vi "traffic control controller.vi"(0 "Is Logging":T3(array[cluster]), 1 "State":u16(ring) items=["Init", "Write"], 5 "Avalanch Packets":T2(array[cluster]) {"A1 std" format="%.1f"; "A2 std" format="%.1f"; "A3 std" format="%.1g"; "A4 std" format="%.1g"}, 13 "Trafikkontroll terskelverdier":T1(array[cluster])) -> (4 "Rød mast":bool[](array[boolean]), 10 "num pack rød lys i sekvens":u16[](array[numeric]), 14 "Is Logging":bool[](array[boolean]))   [LabVIEW 2017]
panel:
  out "num pack rød lys i totalt":u16[](array[numeric])
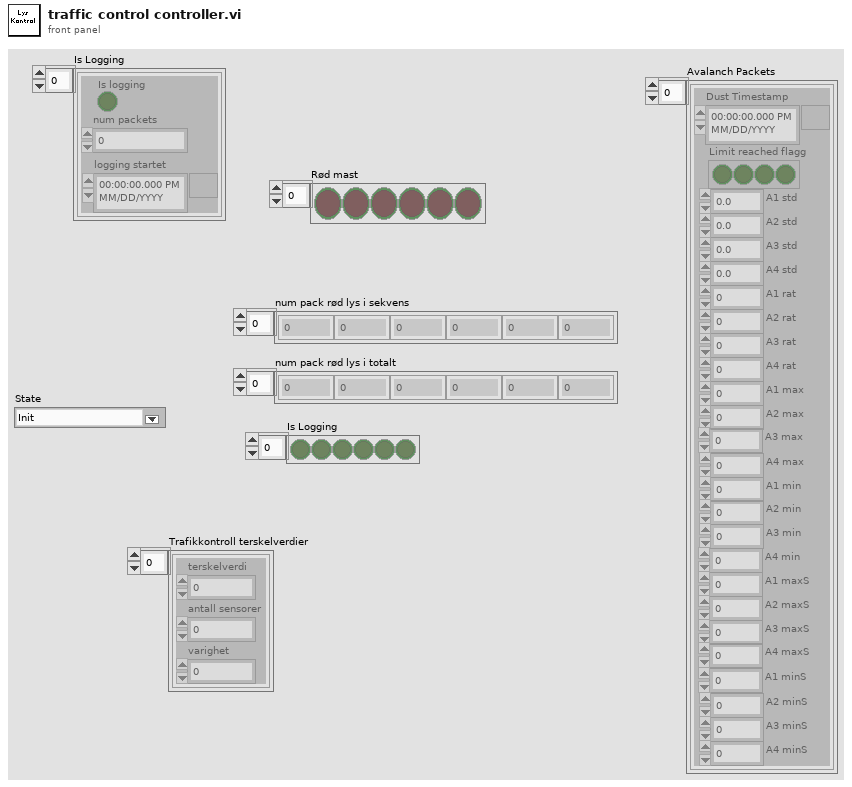
[diagram p1: front panel]
types:
  T1 = cluster{"terskelverdi":u32, "antall sensorer":u32, "varighet":u32}[]
  T2 = cluster{"Dust Timestamp":timestamp, "Limit reached flagg":bool[], "A1 std":sgl, "A2 std":sgl, "A3 std":sgl, "A4 std":sgl, "A1 rat":sgl, "A2 rat":sgl, "A3 rat":sgl, "A4 rat":sgl, "A1 max":u16, "A2 max":u16, "A3 max":u16, "A4 max":u16, "A1 min":u16, "A2 min":u16, "A3 min":u16, "A4 min":u16, "A1 maxS":u16, "A2 maxS":u16, "A3 maxS":u16, "A4 maxS":u16, "A1 minS":u16, "A2 minS":u16, "A3 minS":u16, "A4 minS":u16}[]
  T3 = cluster{"Is logging":bool, "num packets":u16, "logging startet":timestamp}[]
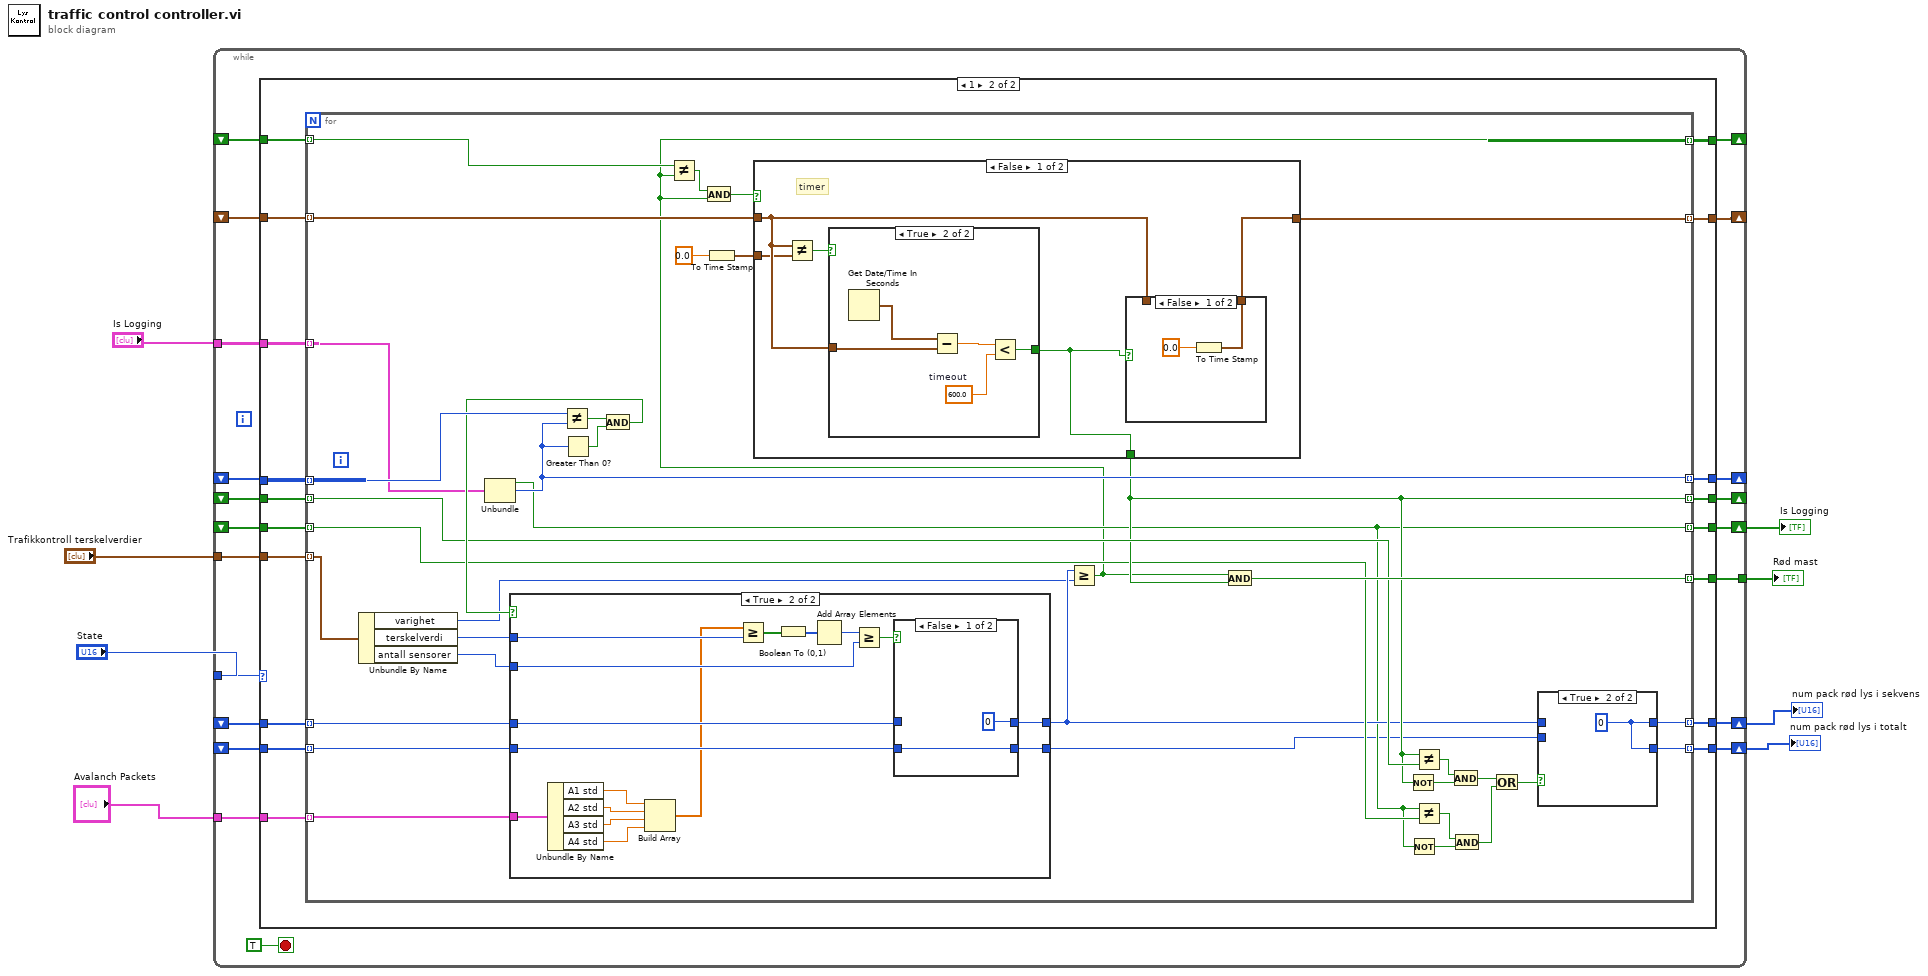
[diagram p0: block diagram]
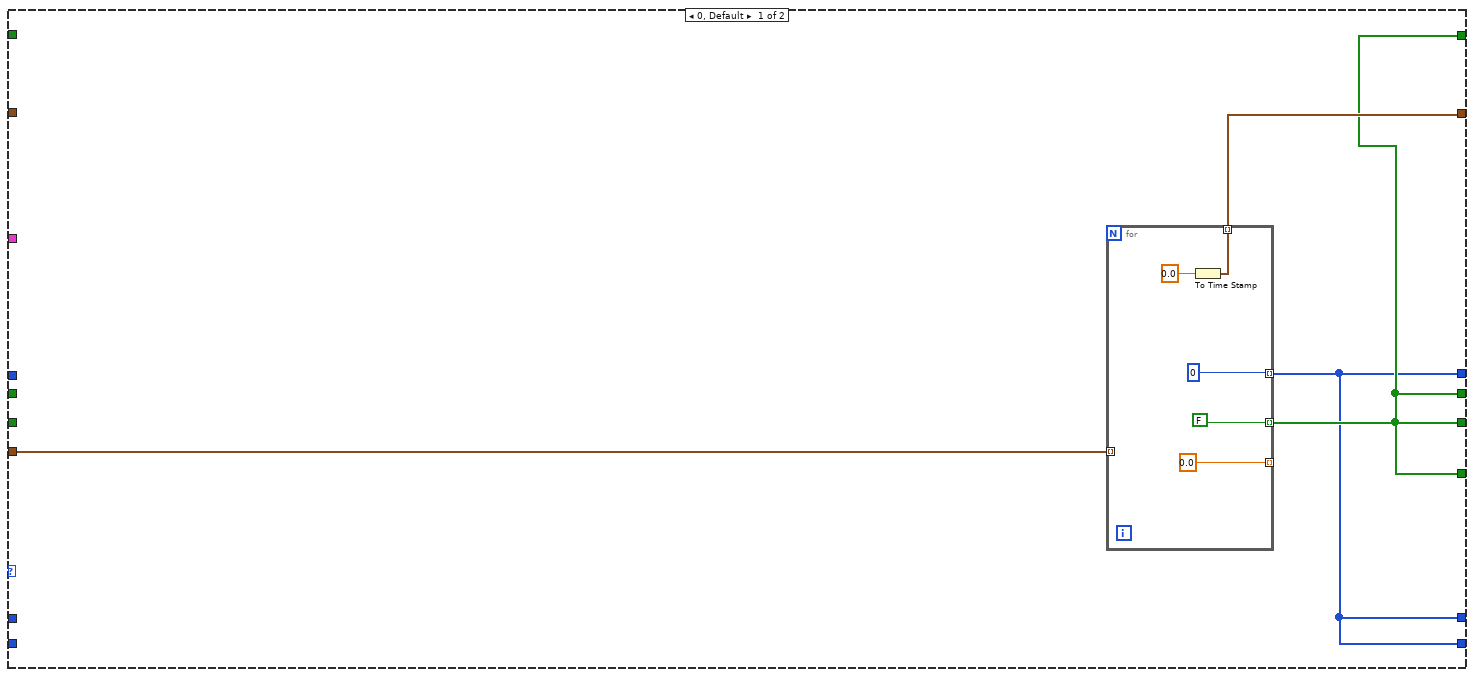
[diagram p2: hidden frame]
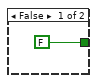
[diagram p5: hidden frame]
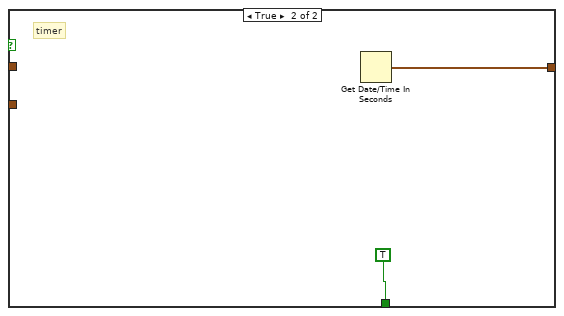
[diagram p6: hidden frame]
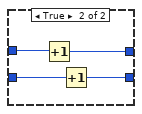
[diagram p8: hidden frame]
diagram:
  n1 = while {
    tunnel: "Is Logging" -> [w28]
    shift-right: [w26] -> _
    shift-left: _ -> [w25]
    tunnel: "Avalanch Packets" -> [w24]
    tunnel: "State" -> [w23]
    shift-right: [w22] -> w6
    shift-left: _ -> [w21]
    shift-right: [w20] -> _
    shift-left: _ -> [w19]
    shift-right: [w18] -> _
    shift-left: _ -> [w17]
    tunnel: [w16] -> w5
    shift-right: [w15] -> _
    shift-left: _ -> [w13]
    shift-right: [w14] -> w4
    shift-left: _ -> [w12]
    shift-right: [w10] -> w2
    shift-left: _ -> [w11]
    tunnel: "Trafikkontroll terskelverdier" -> [w9]
    stop <- TRUE stop-if-true
    n2 = case shown="1" w23 {
      tunnel: w28 -> [_ w55]
      tunnel: [w31 w49] -> w16
      tunnel: [w30 w54] -> w26
      tunnel: w25 -> [_ w53]
      tunnel: w24 -> [_ w52]
      tunnel: [w30 w51] -> w22
      tunnel: w21 -> [_ w50]
      tunnel: [w31 w48] -> w20
      tunnel: w19 -> [_ w47]
      tunnel: [w32 w46] -> w18
      tunnel: w17 -> [_ w45]
      tunnel: [w31 w44] -> w15
      tunnel: [w31 w39] -> w14
      tunnel: w13 -> [_ w43]
      tunnel: w12 -> [_ w42]
      tunnel: w11 -> [_ w41]
      tunnel: [w30 w40] -> w10
      tunnel: w9 -> [w29 w38]
      frame 0, Default {
        n3 = for {
          tunnel: [u16 0] -> w30 mode=indexing
          tunnel: [FALSE] -> w31 mode=indexing
          tunnel: [w34] -> w32 mode=indexing
          tunnel: [0.0 ("number")] -> _ mode=indexing
          tunnel: w29 -> [_] mode=indexing
          n4 = To Time Stamp(1:0.0 ("number")) -> (0:w34:timestamp)
        }
      }
      frame 1 {
        n5 = for {
          tunnel: [w79] -> w49 mode=indexing
          tunnel: w55 -> [w80] mode=indexing
          tunnel: [w86] -> w54 mode=indexing
          tunnel: w53 -> [w92] mode=indexing
          tunnel: w52 -> [w90] mode=indexing
          tunnel: [w69] -> w51 mode=indexing
          tunnel: w50 -> [w87] mode=indexing
          tunnel: [w60] -> w48 mode=indexing
          tunnel: w47 -> [w84] mode=indexing
          tunnel: [w82] -> w46 mode=indexing
          tunnel: w45 -> [w81] mode=indexing
          tunnel: [w75] -> w44 mode=indexing
          tunnel: [w62] -> w39 mode=indexing
          tunnel: w43 -> [w76] mode=indexing
          tunnel: w42 -> [w72] mode=indexing
          tunnel: w41 -> [w64] mode=indexing
          tunnel: [w63] -> w40 mode=indexing
          tunnel: w38 -> [w59] mode=indexing
          n6 = Unbundle By Name(w59) -> ("varighet"=w58:u32, "terskelverdi"=w57:u32, "antall sensorer"=w56:u32)
          n7 = Unbundle(w80) -> ("Is logging"=w62:bool, "num packets"=w86:u16)  [unwired: 1 out]
          n8 = Not Equal?(x=w92, y=w86) -> (x != y?=w91:bool)
          n9 = Greater Than 0?(x=w86) -> (x > 0?=w88:bool)
          n10 = And(x=w91, y=w88) -> (x .and. y?=w89:bool)
          n11 = case shown="True" w89 {
            tunnel: w90 -> [_ w129]
            tunnel: [w113 w120] -> w68
            tunnel: w87 -> [w113 w117]
            tunnel: w56 -> [_ w118]
            tunnel: w57 -> [_ w119]
            tunnel: w64 -> [w112 w116]
            tunnel: [w112 w115] -> w61
            frame False {
            }
            frame True {
              n12 = Unbundle By Name(w129) -> ("A1 std"=w127:sgl, "A2 std"=w128:sgl, "A3 std"=w126:sgl, "A4 std"=w125:sgl)
              n13 = Build Array(w127, w128, w126, w125) -> (w114:sgl[])
              n14 = Greater Or Equal?(x=w114, y=w119) -> (x >= y?=w124:bool[])
              n15 = Boolean To (0,1)(Boolean=w124) -> (0, 1=w123:i16[])
              n16 = Add Array Elements(numeric array=w123) -> (sum=w122:i16)
              n17 = Greater Or Equal?(x=w122, y=w118) -> (x >= y?=w121:bool)
              n18 = case shown="False" w121 {
                tunnel: w117 -> [_ w135]
                tunnel: [u16 0 w134] -> w120
                tunnel: w116 -> [w131 w133]
                tunnel: [w131 w132] -> w115
                frame False {
                }
                frame True {
                  n19 = Increment(x=w135) -> (x+1=w134:u16)
                  n20 = Increment(x=w133) -> (x+1=w132:u16)
                }
              }
            }
          }
          n21 = To Time Stamp(1:0.0 ("number")) -> (0:w66:timestamp)
          n22 = Greater Or Equal?(x=w68, y=w58) -> (x >= y?=w60:bool)
          n23 = Not Equal?(x=w84, y=w60) -> (x != y?=w85:bool)
          n24 = And(x=w85, y=w60) -> (x .and. y?=w83:bool)
          n25 = case shown="False" w83 {
            tunnel: [w100 w111] -> w82
            tunnel: w81 -> [w98 _]
            tunnel: [w96 TRUE] -> w75
            tunnel: w66 -> [w97 _]
            frame False {
              # "timer"
              n26 = Not Equal?(x=w98, y=w97) -> (x != y?=w99:bool)
              n27 = case shown="True" w99 {
                tunnel: w98 -> [_ w109]
                tunnel: [FALSE w106] -> w96
                frame False {
                }
                frame True {
                  w105 = 600.0  # timeout
                  n28 = Get Date/Time In Seconds() -> (seconds since 1Jan1904=w108:timestamp)
                  n29 = Subtract(x=w108, y=w109) -> (x-y=w107:dbl)
                  n30 = Less?(x=w107, y=w105) -> (x < y?=w106:bool)
                }
              }
              n31 = case shown="False" w96 {
                tunnel: [w101 w103] -> w100
                tunnel: w98 -> [_ w103]
                frame False {
                  n32 = To Time Stamp(1:0.0 ("number")) -> (0:w101:timestamp)
                }
                frame True {
                }
              }
            }
            frame True {
              # "timer"
              n33 = Get Date/Time In Seconds() -> (seconds since 1Jan1904=w111:timestamp)
            }
          }
          n34 = And(x=w60, y=w75) -> (x .and. y?=w79:bool)
          n35 = Not(x=w75) -> (.not. x?=w78:bool)
          n36 = Not(x=w62) -> (.not. x?=w74:bool)
          n37 = Not Equal?(x=w75, y=w76) -> (x != y?=w77:bool)
          n38 = Not Equal?(x=w62, y=w72) -> (x != y?=w73:bool)
          n39 = And(x=w77, y=w78) -> (x .and. y?=w71:bool)
          n40 = And(x=w73, y=w74) -> (x .and. y?=w67:bool)
          n41 = Or(x=w71, y=w67) -> (x .or. y?=w70:bool)
          n42 = case shown="True" w70 {
            tunnel: [w94 w95] -> w69
            tunnel: w68 -> [w94 _]
            tunnel: [w93 w95] -> w63
            tunnel: w61 -> [w93 _]
            frame False {
            }
            frame True {
              w95 = u16 0
            }
          }
        }
      }
    }
  }
  "Rød mast" <- w5
  "num pack rød lys i sekvens" <- w6
  "Is Logging" <- w4
  "num pack rød lys i totalt" <- w2
